vi "Client.vi"() -> ()   [LabVIEW 2020]
uses:
  <vilib>/DatastreamGrpc/DatastreamGrpc.lvlib
panel:
  out "#Events":i32
  in  "stop":bool
  out "String":string
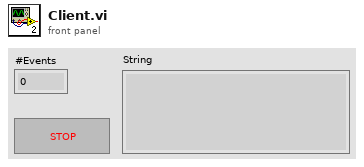
[diagram p1: front panel]
types:
  T1 = typedef "DatastreamGrpc.lvlib/ClientRef.ctl" = cluster{"id":u64}
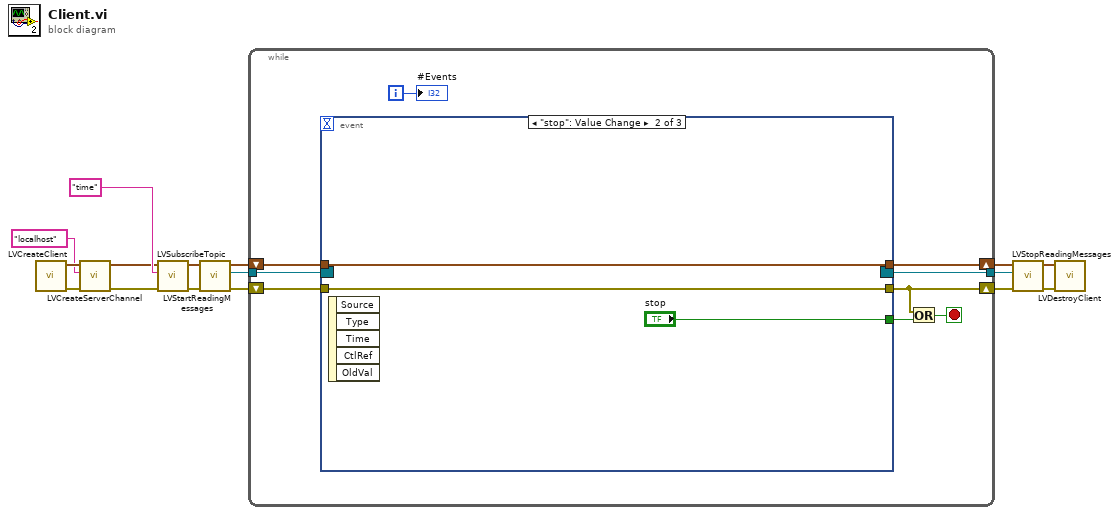
[diagram p0: block diagram]
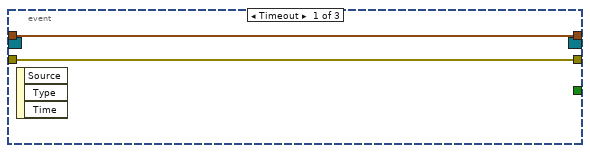
[diagram p2: hidden frame]
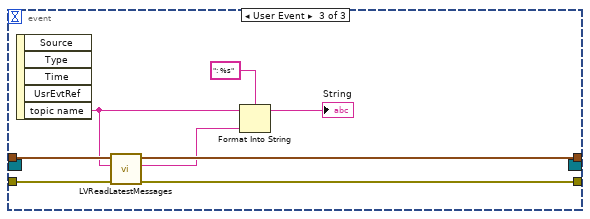
[diagram p3: hidden frame]
diagram:
  n1 = call <vilib>:"LVCreateClient.vi"() -> ("error out"=w9:errorcluster, "ClientRef"=w10:T1)  [unwired: 10 in]
  n2 = call <vilib>:"LVCreateServerChannel.vi"("error in (no error)"=w9, "Server Address"="localhost", "ClientRef in"=w10) -> ("error out"=w8:errorcluster, "ClientRef out"=w1:T1)  [unwired: 7 in]
  n3 = call <vilib>:"LVSubscribeTopic.vi"("error in (no error)"=w8, "Topic to subscribe"="time", "ClientRef in"=w1) -> ("error out"=w3:errorcluster, "ClientRef out"=w4:T1)  [unwired: 7 in]
  n4 = call <vilib>:"LVStartReadingMessages.vi"("error in (no error)"=w3, "ClientRef in"=w4) -> ("error out"=w15:errorcluster, "Event Registration Refnum"=w16:refnum<event-registration>, "ClientRef out"=w2:T1)  [unwired: 7 in]
  n5 = while {
    tunnel: w16 -> [w25]
    shift-right: [w24] -> w13
    shift-left: w2 -> [w23]
    shift-right: [w20] -> w12
    shift-left: w15 -> [w22]
    tunnel: [w18] -> w14
    i -> [w17]
    stop <- w19 stop-if-true
    n6 = event shown="[1] \"stop\": Value Change" {
      selector: w25 -> [_ _ _]
      dyn-events: [_ _ _] -> w18
      timeout: _ -> [_ _ _]
      tunnel: [w27 w28 w36] -> w24
      tunnel: w23 -> [w27 w28 w38]
      tunnel: [w26 w30 w35] -> w20
      tunnel: w22 -> [w26 w30 w37]
      tunnel: [_ "stop" _] -> w21
      event Timeout {
        n7 = event-data() -> ()  [unwired: 1 in, 3 out]
      }
      event "stop": Value Change {
        n8 = event-data() -> ()  [unwired: 1 in, 5 out]
      }
      event User Event {
        n9 = event-data() -> ("topic name"=w34:string)  [unwired: 1 in, 4 out]
        n10 = call <vilib>:"LVReadLatestMessages.vi"("error in (no error)"=w37, "Subscribed Topic"=w34, "ClientRef in"=w38) -> ("error out"=w35:errorcluster, "Topic message data out"=w32:string, "ClientRef out"=w36:T1)  [unwired: 6 in]
        n11 = Format Into String(format string=": %s", initial string=w34, w32) -> (resulting string=→"String":string)  [unwired: 1 in, 1 out]
      }
    }
    n12 = Or(x=w20, y=w21) -> (x .or. y?=w19:bool)
    "#Events" <- w17
  }
  n13 = call <vilib>:"LVStopReadingMessages.vi"("error in (no error)"=w12, "Event Registration Refnum"=w14, "ClientRef in"=w13) -> ("error out"=w6:errorcluster, "ClientRef out"=w5:T1)  [unwired: 7 in]
  n14 = call <vilib>:"LVDestroyClient.vi"("error in (no error)"=w6, "ClientRef"=w5) -> ()  [unwired: 9 in, 1 out]
